vi "Modeshift Control.vi"(0 "GEA2 Reference In":refnum<k24>, 5 "Shift To":enum16{"Spin", "Agitate"}(ring), 11 "Error In":errorcluster) -> (4 "GEA2 Reference Out":refnum<k24>, 6 "Pass/Fail?":bool, 8 "Report Text":string, 15 "Error Out":errorcluster)   [LabVIEW 2016, in "TL27.lvlib"]
doc: "Use this VI to request a modeshift."
uses:
  Projects/TL27.lvlib
  C:/Automation/DLLs/PC Dot Net/GeaCommunication.dll
  Common/LabVIEW GEA2 Toolkit/LabVIEW_GEA2_Toolkit.lvlibp/type defs/Source_Destination.ctl
  Common/LabVIEW GEA2 Toolkit/LabVIEW_GEA2_Toolkit.lvlibp/type defs/ERD Read Data In.ctl
  Common/LabVIEW GEA2 Toolkit/LabVIEW_GEA2_Toolkit.lvlibp/type defs/Data Type.ctl
  Common/LabVIEW GEA2 Toolkit/LabVIEW_GEA2_Toolkit.lvlibp/type defs/ERD Write Data In.ctl
  Common/LabVIEW GEA2 Toolkit/LabVIEW_GEA2_Toolkit.lvlibp
panel:
  in  "Standalone?":bool
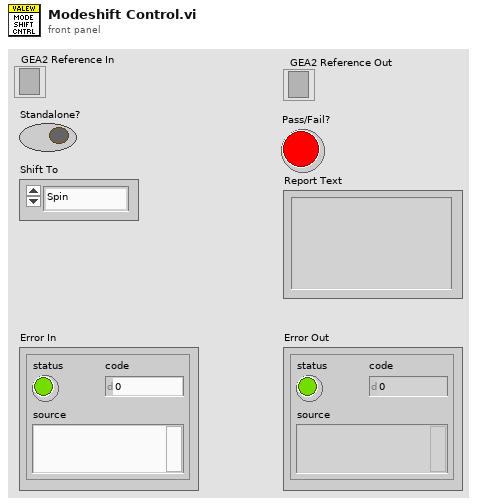
[diagram p1: front panel]
types:
  T1 = enum16{"EQ (==)", "NE (!=)", "GT (>)", "LT (<)", "GE (>=)", "LE (<=)", "GTLT(> <)", "GELE (>= <=)", "GELT (>= <)", "GTLE (> <=)", "LTGT (< >)", "LEGE (<= >=)", "LEGT (<= >)", "LTGE (< >=)", "No Comparison"}
  T2 = typedef "LabVIEW_GEA2_Toolkit.lvlibp/ERD Read Data In.ctl" = cluster{"ERD Number":u16, "Data Type":T3}
  T3 = typedef "LabVIEW_GEA2_Toolkit.lvlibp/Data Type.ctl" = enum16{"string", "boolean", "uint8_t", "uint16_t", "uint32_t", "uint64_t", "int8_t", "int16_t", "int32_t", "int64_t"}
  T4 = typedef "LabVIEW_GEA2_Toolkit.lvlibp/Source_Destination.ctl" = cluster{"Source":u8, "Destination":u8}
  T5 = typedef "LabVIEW_GEA2_Toolkit.lvlibp/ERD Write Data In.ctl" = cluster{"ERD Number":u16, "Data Type":T3, "Data":string}
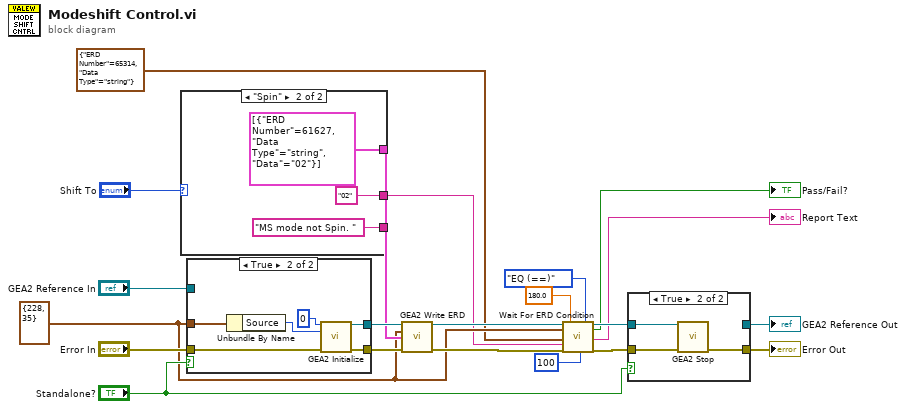
[diagram p0: block diagram]
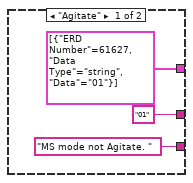
[diagram p2: hidden frame]
diagram:
  w11 = T4 {"Source"=228, "Destination"=35} ("GEA Inputs")
  n1 = case shown="\"Spin\"" "Shift To" {
    tunnel: [T5[] [{"ERD Number"=61627, "Data Type"=enum."string", "Data"="01"}] ("Write ERD List") T5[] [{"ERD Number"=61627, "Data Type"=enum."string", "Data"="02"}] ("Write ERD List")] -> w14
    tunnel: ["01" ("y") "02" ("y")] -> w6
    tunnel: ["MS mode not Agitate. " ("f") "MS mode not Spin. " ("f")] -> _
    frame "Agitate" {
    }
    frame "Spin" {
    }
  }
  n2 = case shown="True" "Standalone?" {
    tunnel: "Error In" -> [w28 w35]
    tunnel: [w28 w34] -> w15
    tunnel: "GEA2 Reference In" -> [w29 _]
    tunnel: [w29 w33] -> w21
    tunnel: w11 -> [_ w31]
    frame False {
    }
    frame True {
      n3 = Unbundle By Name(w31) -> ("Source"=w32:u8)
      n4 = call "GEA2 Initialize.vi"("Board Index"=0, "Source Address"=w32, "error in"=w35) -> ("GEA2 Reference Out"=w33:refnum<k24>, "error out"=w34:errorcluster)  [unwired: 10 in, 1 out]
    }
  }
  n5 = call "GEA2 Write ERD.vi"("GEA2 Reference In"=w21, "GEA Inputs"=w11, "Write ERD List"=w14, "Error In"=w15) -> ("GEA2 Reference Out"=w13:refnum<k24>, "Error Out"=w12:errorcluster)  [unwired: 9 in, 1 out]
  n6 = call "Wait For ERD Condition.vi"("GEA2 Reference In"=w13, "GEA Inputs"=w11, "ERD Read Data"=T2 {"ERD Number"=65314, "Data Type"=enum."string"} ("ERD Read Data In"), "Expected Low"=w6, "Error In"=w12, "Timeout (s)"=180.0, "Loop Rate (ms)"=u32 100, "Comparison"=T1."EQ (==)") -> ("GEA2 Reference Out"=w10:refnum<k24>, "Pass/Fail?"=→"Pass/Fail?":bool, "Report Text"=→"Report Text":string, "Error Out"=w9:errorcluster)  [unwired: 7 in, 1 out]
  n7 = case shown="True" "Standalone?" {
    tunnel: w9 -> [w37 w40]
    tunnel: [w37 w39] -> w20
    tunnel: [w36 _] -> w19
    tunnel: w10 -> [w36 w38]
    frame False {
    }
    frame True {
      n8 = call "GEA2 Stop.vi"("GEA2 Reference In"=w38, "Error In"=w40) -> ("Error Out"=w39:errorcluster)  [unwired: 13 in]
    }
  }
  "Error Out" <- w20
  "GEA2 Reference Out" <- w19
